vi "One.vi"(8 "error in (no error)":errorcluster, 11 "Mock in":refnum<class "Mock.lvclass">) -> (0 "error out":errorcluster, 3 "Mock out":refnum<class "Mock.lvclass">)   [LabVIEW 2020, in "One.lvclass"]
uses:
  One Of/One.lvclass
  Mock.lvclass
  C:/git/astemes-lmock/sandbox/Expectation/Expectation.lvclass
  One Of/One.lvclass/One.ctl
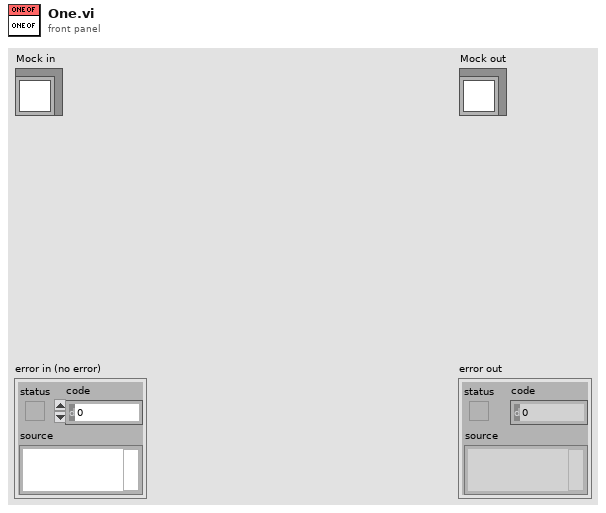
[diagram p1: front panel]
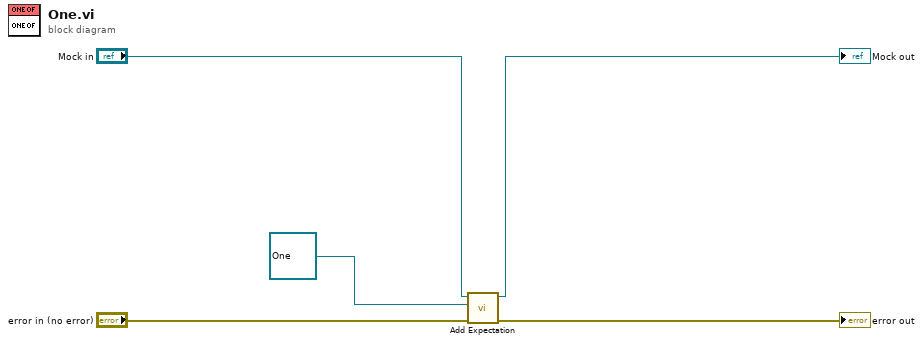
[diagram p0: block diagram]
diagram:
  n1 = call "Add Expectation.vi"("error in (no error)"="error in (no error)", "Expectations"=refnum<class "One.lvclass"> refnum ("One Of.lvclass"), "Mock in"="Mock in") -> ("error out"=→"error out":errorcluster, "Mock out"=→"Mock out":refnum<class "Mock.lvclass">)  [unwired: 7 in]
